vi "inverse Kinematics.vi"(6 "constant":cluster{"d1":dbl, "a2":dbl, "a3":dbl}={"d1"=100.0, "a2"=67.0, "a3"=120.0}, 9 "Pz":dbl, 10 "Py":dbl, 11 "Px":dbl) -> (1 "theta3a":dbl, 2 "theta2a":dbl, 3 "theta1a":dbl)   [LabVIEW 2017]
uses:
  <vilib>/imath/engines/lvmath2/RunTimeEngine/BuiltInFunctions/atan2/NIMS_atan2.vi
  <instcachedir>/0/NIMS_atan2_A91AA4A7D42247EDBE8F76DB99AF04A4.lvgen/NIMS_atan2_A91AA4A7D42247EDBE8F76DB99AF04A4_000.vi
  <vilib>/imath/engines/lvmath2/RunTimeEngine/BuiltInFunctions/cos/NIMS_cos(C).vi
  <instcachedir>/0/NIMS_cos(C)_D76AB42705D04DD7AB90183D51B32C21.lvgen/NIMS_cos(C)_D76AB42705D04DD7AB90183D51B32C21_001.vi
  <vilib>/imath/engines/lvmath2/RunTimeEngine/BuiltInFunctions/sin/NIMS_sin(C).vi
  <instcachedir>/0/NIMS_sin(C)_3AEF00A0D47841AA8A3F5FC7392BEEFD.lvgen/NIMS_sin(C)_3AEF00A0D47841AA8A3F5FC7392BEEFD_001.vi
  <vilib>/imath/engines/lvmath2/RunTimeEngine/ArithmeticOperatorToken/NIMS_ArithmeticOperator_power(S).vi
  <instcachedir>/0/NIMS_ArithmeticOperator_power(S)_86B1D76B77564424912EAFCCCC7488ED.lvgen/NIMS_ArithmeticOperator_power(S)_86B1D76B77564424912EAFCCCC7488ED_010.vi
  <vilib>/imath/engines/lvmath2/RunTimeEngine/BuiltInFunctions/atan/NIMS_atan(C).vi
  <instcachedir>/0/NIMS_atan(C)_1FAE31362B334AE8BEB442177AE08699.lvgen/NIMS_atan(C)_1FAE31362B334AE8BEB442177AE08699_001.vi
  <instcachedir>/0/NIMS_ArithmeticOperator_power(S)_86B1D76B77564424912EAFCCCC7488ED.lvgen/NIMS_ArithmeticOperator_power(S)_86B1D76B77564424912EAFCCCC7488ED_009.vi
  <vilib>/imath/engines/lvmath2/RunTimeEngine/BuiltInFunctions/asin/NIMS_asin(C).vi
  <instcachedir>/0/NIMS_asin(C)_AC3BFCB47B1546A49EF59786BF54013C.lvgen/NIMS_asin(C)_AC3BFCB47B1546A49EF59786BF54013C_001.vi
  <vilib>/imath/engines/lvmath2/RunTimeEngine/ErrorHandling/NIMS_Create Error From Enums.vi
  <vilib>/imath/engines/lvmath2/RunTimeEngine/NodeEndStatement/NIMS_NodeEndStatement_Output.vi
  <instcachedir>/0/NIMS_NodeEndStatement_Output_53EC0D466D134D7ABD903AC30B43404B.lvgen/NIMS_NodeEndStatement_Output_53EC0D466D134D7ABD903AC30B43404B_009.vi
  <instcachedir>/0/NIMS_NodeEndStatement_Output_53EC0D466D134D7ABD903AC30B43404B.lvgen/NIMS_NodeEndStatement_Output_53EC0D466D134D7ABD903AC30B43404B_001.vi
  <vilib>/imath/engines/lvmath2/RunTimeEngine/ErrorHandling/NIMS_Finalize Error.vi
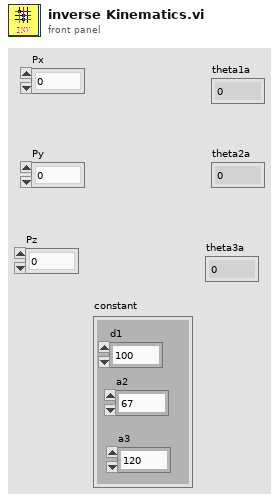
[diagram p1: front panel]
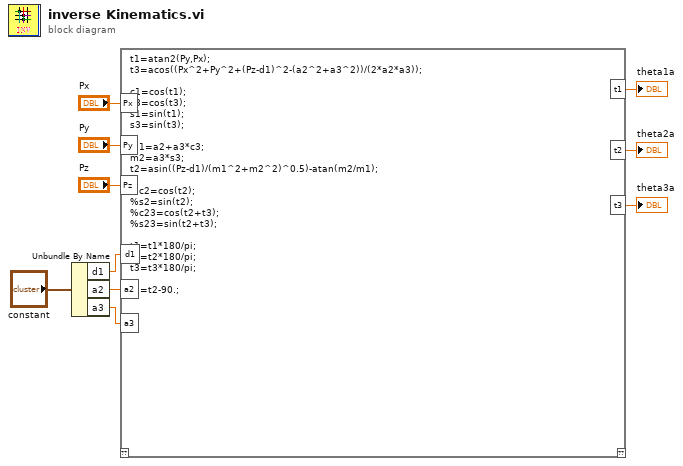
[diagram p0: block diagram]
diagram:
  n1 = Unbundle By Name("constant") -> ("d1"=w9:dbl, "a2"=w8:dbl, "a3"=w7:dbl)
  n2 = mathscript code="t1=atan2(Py,Px);\nt3=acos((Px^2+Py^2+(Pz-d1)^2-(a2^2+a3^2))/(2*a2*a3));\n\nc1=cos(t1);\nc3=cos(t3);\ns1=sin(t1);\ns3=sin(t3);\n\nm1=a2+a3*c3;\nm2=a3*s3;\nt2=asin((Pz-d1)/(m1^2+m2^2)^0.5)-atan(m2/m1);\n\n%c2=cos(t2);\n%s2=sin(t2);\n%c23=cos(t2+t3);\n%s23=sin(t2+t3);\n\nt1=t1*180/pi;\nt2=t2*180/pi;\nt3=t3*180/pi;\n\nt2=t2-90.;"("Px"="Px", "Py"="Py", "Pz"="Pz", "d1"=w9, "a2"=w8, "a3"=w7) -> ("t1"=→"theta1a":dbl, "t2"=→"theta2a":cdb, "t3"=→"theta3a":cdb)  [unwired: 1 in, 1 out]
